vi "Arduino_communication_Testcode.vi"() -> ()   [LabVIEW 2022 SP3]
uses:
  <vilib>/Instr/_visa.llb/VISA Find Search Mode.ctl
  fc2f3981-17a7-460f-9bf9-74dae72a1d09.vi
  baeb2f91-fd90-4595-bb3c-d856673473f2.vi
  b76835a7-dad6-4b12-b3e4-a4cb3ce1286a.vi
  da959e76-b1b2-43a4-b05c-2468bb163dc8.vi
  <vilib>/regexp/Match Regular Expression.xnode
panel:
  out "Numeric":i32
  out "Serial Settings:Number of Bytes at Serial Port":u32
  out "read buffer":string
  out "Message counter":i32
  out "Arduino 3":refnum<visa-resource-name>
  in  "stop":bool
  out "Valve state":dbl
  out "error IO":errorcluster
  in  "Close(T)/Open(F)":bool
  out "Array":string[](array[string])
  in  "error in":errorcluster
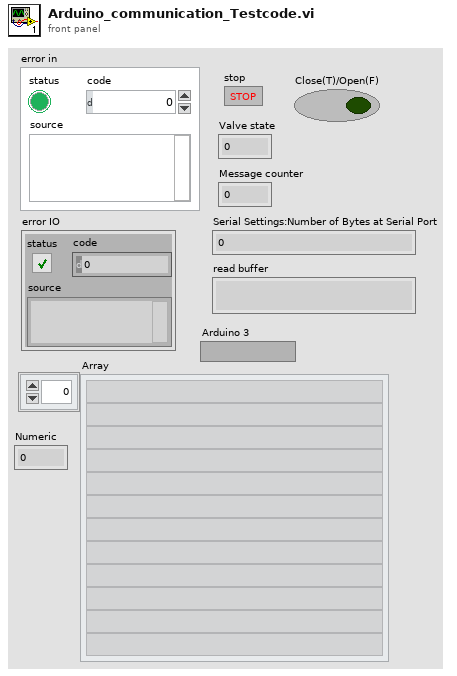
[diagram p1: front panel]
types:
  T1 = cluster{"VISA resource name":refnum<visa-resource-name>, "error out":errorcluster}
  T2 = typedef "VISA Find Search Mode.ctl" = u32
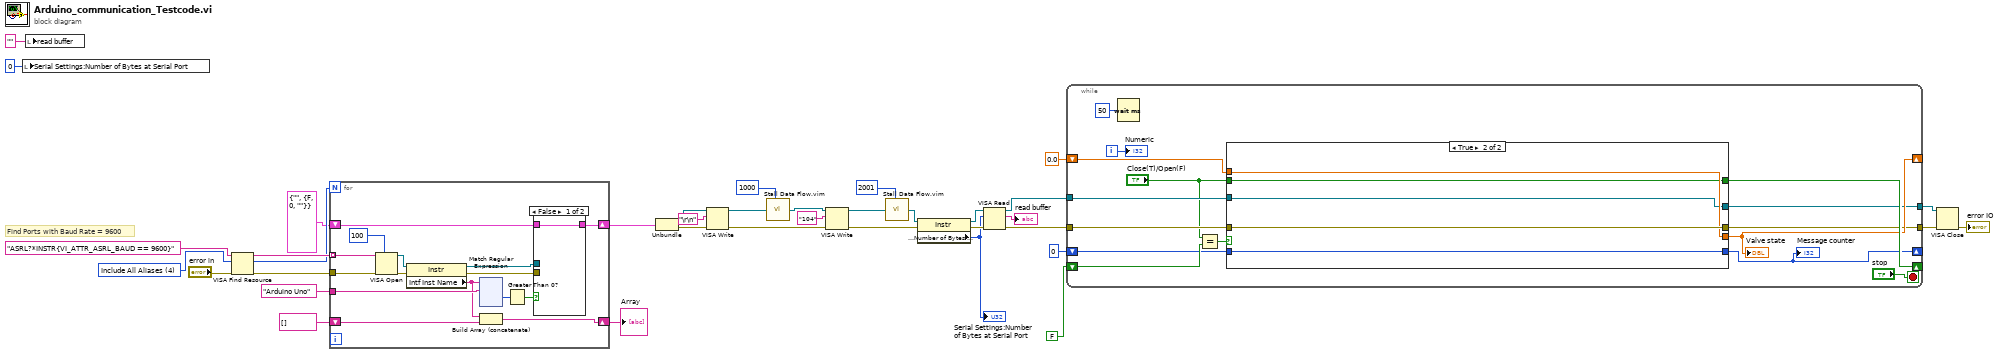
[diagram p0: block diagram]
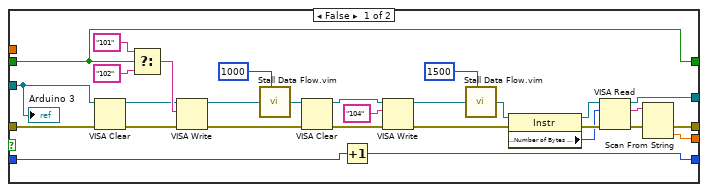
[diagram p2: hidden frame]
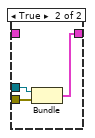
[diagram p3: hidden frame]
diagram:
  w32 = T2 4 items=["Canonical Names Only"=0, "Aliases Only"=2, "Include Matching Aliases"=3, "Include All Aliases"=4] ("Search Mode")
  # "Find Ports with Baud Rate = 9600"
  n1 = local write "Serial Settings:Number of Bytes at Serial Port"(u32 0 ("Serial Settings:Number of Bytes at Serial Port")) -> ()
  n2 = local write "read buffer"("" ("read buffer")) -> ()
  n3 = VISA Find Resource(8:"error in", 10:w32, 11:"ASRL?*INSTR{VI_ATTR_ASRL_BAUD == 9600}" ("expression (\"?*\")")) -> (0:w34:errorcluster, 2:w29:u32, 3:w37:string[])
  n4 = for {
    N: w29 -> [_]
    tunnel: w37 -> [w52] mode=indexing
    tunnel: "Arduino Uno" -> [w48]
    shift-right: [w46] -> w36
    shift-left: T1 {"VISA resource name"="", "error out"={"status"=FALSE, "code"=0, "source"=""}} -> [w45]
    tunnel: w34 -> [w44]
    shift-right: [w39] -> w28
    shift-left: string[] [] -> [w38]
    n5 = VISA Open(timeout (0)=u32 100 ("VISA Open timeout (0)"), error in (no error)=w44, VISA resource name=w52) -> (VISA resource name=w51:refnum<visa-resource-name>, error out=w47:errorcluster)  [unwired: 2 in]
    n6 = property class="Instr"(reference=w51, error in=w47) -> (reference out=w43:refnum<visa-resource-name>, error out=w42:errorcluster, "Intf Inst Name"=w40:string)
    n7 = xnode "Match Regular Expression"("input string"=w40, "regular expression"=w48) -> ("offset past match"=w50:i32)  [unwired: 4 in, 4 out]
    n8 = Build Array (concatenate)(w40, w38) -> (w39:string[])
    n9 = Greater Than 0?(x=w50) -> (x > 0?=w49:bool)
    n10 = case shown="False" w49 {
      tunnel: w43 -> [_ w56]
      tunnel: w42 -> [_ w55]
      tunnel: [w53 w54] -> w46
      tunnel: w45 -> [w53 _]
      frame False {
      }
      frame True {
        n11 = Bundle("VISA resource name"=w56, "error out"=w55) -> (w54:T1)  [unwired: 1 in]
      }
    }
  }
  "Array" <- w28
  n12 = Unbundle(w36) -> ("VISA resource name"=w7:refnum<visa-resource-name>, "error out"=w6:errorcluster)
  n13 = VISA Write(VISA resource name=w7, write buffer="\r\n", error in (no error)=w6) -> (VISA resource name out=w18:refnum<visa-resource-name>, error out=w16:errorcluster)  [unwired: 1 out]
  n14 = call "Stall Data Flow.vim"("value in"=w18, "milliseconds to wait"=u32 1000) -> ("value out"=w17:refnum<visa-resource-name>)  [unwired: 1 out]
  n15 = VISA Write(VISA resource name=w17, write buffer="104", error in (no error)=w16) -> (VISA resource name out=w25:refnum<visa-resource-name>, error out=w24:errorcluster)  [unwired: 1 out]
  n16 = call "Stall Data Flow.vim"("value in"=w25, "milliseconds to wait"=u32 2001) -> ("value out"=w26:refnum<visa-resource-name>)  [unwired: 1 out]
  n17 = property class="Instr"(reference=w26, error in=w24) -> (reference out=w22:refnum<visa-resource-name>, error out=w23:errorcluster, "Serial Settings:Number of Bytes at Serial Port"=w19:u32)
  "Serial Settings:Number of Bytes at Serial Port" <- w19
  n18 = VISA Read(VISA resource name=w22, byte count=w19, error in (no error)=w23) -> (VISA resource name out=w14:refnum<visa-resource-name>, read buffer=→"read buffer":string, error out=w13:errorcluster)  [unwired: 1 out]
  n19 = while {
    tunnel: w14 -> [w188]
    tunnel: w13 -> [w187]
    shift-right: [w185] -> _
    shift-left: FALSE ("Close(T)/Open(F)") -> [w182]
    shift-right: [w181] -> _
    shift-left: 0.0 -> [w180]
    shift-right: [w177] -> _
    shift-left: 0 -> [w178]
    tunnel: [w175] -> w3
    tunnel: [w174] -> w2
    i -> [w176]
    stop <- "stop" stop-if-true
    n20 = Wait (ms)(milliseconds to wait=u32 50) -> ()  [unwired: 1 out]
    n21 = Equal?(x="Close(T)/Open(F)", y=w182) -> (x = y?=w184:bool)
    n22 = case shown="True" w184 {
      tunnel: w188 -> [w191 w218]
      tunnel: w187 -> [w190 w222]
      tunnel: [w195 w221] -> w181
      tunnel: [w196 w222] -> w175
      tunnel: "Close(T)/Open(F)" -> [w197 w220]
      tunnel: [w197 w220] -> w185
      tunnel: w180 -> [_ w221]
      tunnel: w178 -> [w193 w219]
      tunnel: [w192 w219] -> w177
      tunnel: [w189 w218] -> w174
      frame False {
        n23 = VISA Clear(VISA resource name=w191, error in (no error)=w190) -> (VISA resource name out=w205:refnum<visa-resource-name>, error out=w207:errorcluster)
        n24 = Select(t="101", s=w197, f="102") -> (s? t:f=w206:string)
        n25 = VISA Write(VISA resource name=w205, write buffer=w206, error in (no error)=w207) -> (VISA resource name out=w208:refnum<visa-resource-name>, error out=w204:errorcluster)  [unwired: 1 out]
        n26 = call "Stall Data Flow.vim"("value in"=w208, "milliseconds to wait"=u32 1000) -> ("value out"=w203:refnum<visa-resource-name>)  [unwired: 1 out]
        n27 = VISA Clear(VISA resource name=w203, error in (no error)=w204) -> (VISA resource name out=w215:refnum<visa-resource-name>, error out=w216:errorcluster)
        n28 = Increment(x=w193) -> (x+1=w192:i32)
        n29 = VISA Write(VISA resource name=w215, write buffer="104", error in (no error)=w216) -> (VISA resource name out=w212:refnum<visa-resource-name>, error out=w211:errorcluster)  [unwired: 1 out]
        n30 = call "Stall Data Flow.vim"("value in"=w212, "milliseconds to wait"=u32 1500) -> ("value out"=w213:refnum<visa-resource-name>)  [unwired: 1 out]
        n31 = property class="Instr"(reference=w213, error in=w211) -> (reference out=w209:refnum<visa-resource-name>, error out=w210:errorcluster, "Serial Settings:Number of Bytes at Serial Port"=w194:u32)
        n32 = VISA Read(VISA resource name=w209, byte count=w194, error in (no error)=w210) -> (VISA resource name out=w189:refnum<visa-resource-name>, read buffer=w217:string, error out=w214:errorcluster)  [unwired: 1 out]
        n33 = Scan From String(input string=w217, error in=w214) -> (error out=w196:errorcluster, output 1=w195:dbl)  [unwired: 3 in, 2 out]
        "Arduino 3" <- w191
      }
      frame True {
      }
    }
    "Valve state" <- w181
    "Message counter" <- w177
    "Numeric" <- w176
  }
  n34 = VISA Close(VISA resource name=w2, error in (no error)=w3) -> (error out=→"error IO":errorcluster)
